vi "Test API Execution from Class Path.vi"(8 "error in (no error)":errorcluster, 11 "API Test in":refnum<class "API Test.lvclass">) -> (0 "error out":errorcluster, 3 "API Test out":refnum<class "API Test.lvclass">)   [LabVIEW 2020, in "LUnit Tests.lvlib" / "API Test.lvclass"]
uses:
  API Test.lvclass
  C:/Program Files (x86)/National Instruments/LabVIEW 2020/vi.lib/Astemes/LUnit/Test Case.lvclass
  Test Dummys/Test Test Case/Test Test Case.lvclass
  <vilib>/Astemes/LUnit/Test Case.lvclass/Test Case.ctl
  <vilib>/Astemes/LUnit/Palette/Fail.vi
  <vilib>/Astemes/LUnit/Palette/Pass.vi
  <vilib>/Astemes/LUnit/Set Assertion Type.vi
  <vilib>/Astemes/LUnit/Add test result.vi
  <vilib>/Astemes/LUnit/LUnit Record Assertion Result.vi
  <vilib>/Astemes/LUnit/LUnit Aggregate Assertion Results.vi
  <vilib>/Astemes/LUnit/Method Result/LUnit Merge Status.vi
  <vilib>/Astemes/LUnit/LUnit Concatenate result strings.vi
  API Test.lvclass/API Test.ctl
  source/Framework/Execution API/Execution API.lvclass
  <vilib>/Astemes/LUnit/Test Case.lvclass
  C:/Git/astemes-lunit/tests/API Test/API Test.lvclass
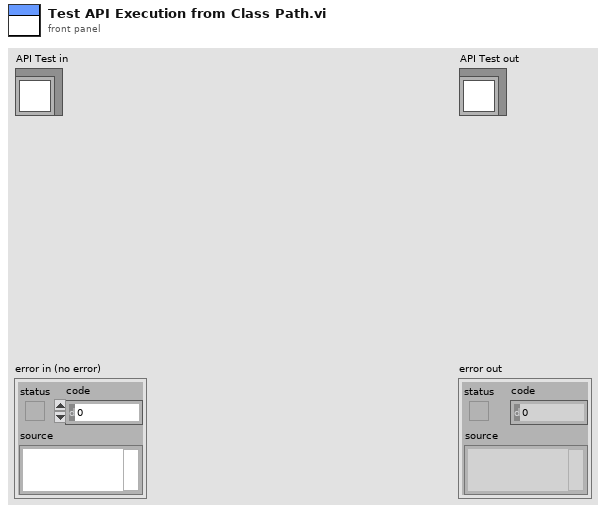
[diagram p1: front panel]
types:
  T1 = cluster{"Result Events":refnum<event-registration>, "Event Registration Refnum":refnum<event-registration>}
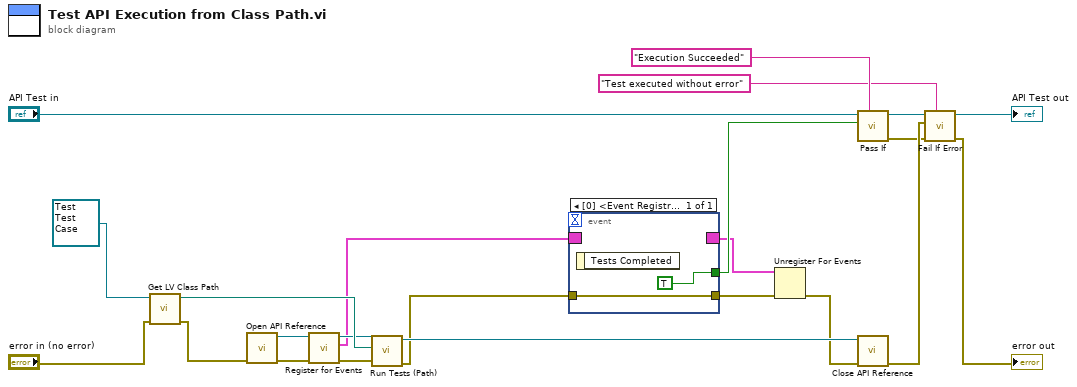
[diagram p0: block diagram]
diagram:
  n1 = call <vilib>:"Get LV Class Path.vi"("error in (no error)"="error in (no error)", "object"=refnum<class "Test Test Case.lvclass"> refnum ("Test Test Case.lvclass")) -> ("error out"=w9:errorcluster, "class path"=w19:path)  [unwired: 8 in]
  n2 = call "Open API Reference.vi"("error in (no error)"=w9) -> ("error out"=w23:errorcluster, "Execution API out"=w3:refnum<class "Execution API.lvclass">)  [unwired: 9 in]
  n3 = call "Register for Events.vi"("error in (no error)"=w23, "Execution API in"=w3) -> ("error out"=w4:errorcluster, "Event Registrations"=w1:T1, "Execution API out"=w2:refnum<class "Execution API.lvclass">)  [unwired: 7 in]
  n4 = call "Run Tests (Path).vi"("error in (no error)"=w4, "Project or Class Path"=w19, "Execution API In"=w2) -> ("error out"=w21:errorcluster, "Execution API Out"=w22:refnum<class "Execution API.lvclass">)  [unwired: 7 in]
  n5 = event shown="[0] <Event Registration Refnum.Test Completed>: User Event" {
    selector: w1 -> [_]
    dyn-events: [_] -> w7
    timeout: _ -> [_]
    tunnel: [TRUE] -> w13
    tunnel: w21 -> [w24]
    tunnel: [w24] -> w6
    event User Event {
      n6 = event-data() -> ()  [unwired: 1 in, 1 out]
    }
  }
  n7 = Unregister For Events(event registration refnum=w7, error in=w6) -> (error out=w8:errorcluster)
  n8 = call <vilib>:"Pass If.vi"("Description"="Execution Succeeded", "Pass?"=w13, "LUnit Test Case In"="API Test in") -> ("error out"=w14:errorcluster, "LUnit Test Case Out"=w15:refnum<class "API Test.lvclass">)  [unwired: 7 in]
  n9 = call "Close API Reference.vi"("error in (no error)"=w8, "Execution API in"=w22) -> ("error out"=w17:errorcluster)  [unwired: 9 in]
  n10 = call <vilib>:"Fail If Error.vi"("Description"="Test executed without error", "error in (no error)"=w14, "Assert error"=w17, "LUnit Test Case In"=w15) -> ("error out"=→"error out":errorcluster, "LUnit Test Case Out"=→"API Test out":refnum<class "API Test.lvclass">)  [unwired: 6 in]
